vi "Read Report Q.vi"(8 "error in (no error)":errorcluster, 11 "Engine in":refnum<class "Engine.lvclass">) -> (0 "error out":errorcluster, 2 "Report Q":refnum<class "QDMH.lvclass">, 3 "Engine out":refnum<class "Engine.lvclass">)   [LabVIEW 2023, in "Engine.lvlib" / "Engine.lvclass"]
uses:
  Library/Engine.lvclass
  Library/Engine.lvclass/Engine.ctl
  builds/Tools/QDMH.lvlibp/Library/QDMH.lvclass
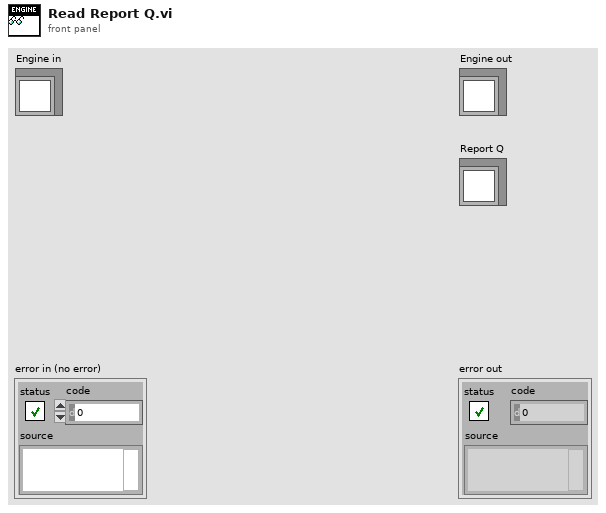
[diagram p1: front panel]
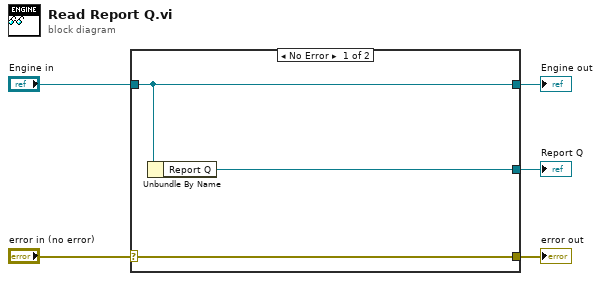
[diagram p0: block diagram]
diagram:
  n1 = case shown="No Error" "error in (no error)" {
    selector: "error in (no error)" -> [w8 w9]
    tunnel: [w8 w9] -> w4
    tunnel: [w7 w10] -> w2
    tunnel: "Engine in" -> [w7 w10]
    tunnel: [w6 _] -> w1
    frame No Error {
      n2 = Unbundle By Name(w7) -> ("Report Q"=w6:refnum<class "QDMH.lvclass">)
    }
    frame Error {
    }
  }
  "error out" <- w4
  "Engine out" <- w2
  "Report Q" <- w1
